vi "Variables Data IO.vi"(6 "Write blank data ?(F)":bool, 7 "Select":T1, 8 "error in":errorcluster caption="에러 입력(에러 없음)", 9 "Data In":string[][](array[string]), 11 "Func_ext":string) -> (0 "error out":errorcluster caption="에러 출력", 1 "Data Out":string[][](array[string]), 3 "Func_ext Out":string)   [LabVIEW 2020]
uses:
  Controls/Cmd_Var Data IO.ctl
  Variables/Global_Condition.vi
  Variables/Global_Resolution.vi
  Variables/Global_Spec.vi
  Variables/Global_Result.vi
  Variables/Global_STD.vi
  Variables/Global_CMC.vi
  Variables/Global_Cal Info.vi
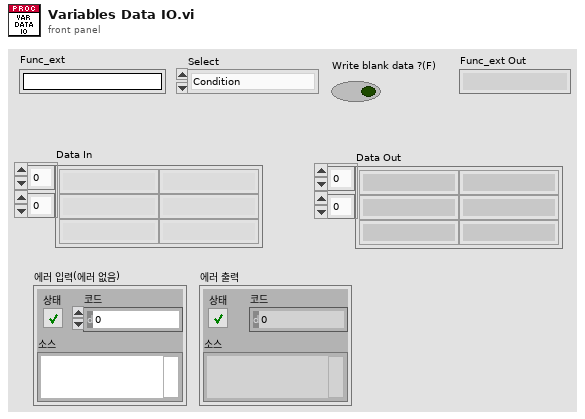
[diagram p1: front panel]
types:
  T1 = typedef "Cmd_Var Data IO.ctl" = enum16{"Condition", "Condition Default", "Condition_Temp", "Resolution", "Resolution Default", "Resolution Old", "Spec", "Spec Default", "Spec Old", "Spec Temp", "Result", "Result2", "Result3", "Result_Temp", "Result_ADJ", "Result_ADJ2", "STD1", "STD2", "STD3", "STD4", "STD5", "STD Temp", "CMC", "CMC Default"}
  T2 = cluster{"Func 0":string[][], "Func 1":string[][], "Func 2":string[][], "Func 3":string[][], "Func 4":string[][], "Func 5":string[][], "Func 6":string[][], "Func 7":string[][], "Func 8":string[][], "Func 9":string[][], "Func 10":string[][], "Func 11":string[][], "Func 12":string[][], "Func 13":string[][], "Func 14":string[][], "Func 15":string[][], "Func 16":string[][], "Func 17":string[][], "Func 18":string[][], "Func 19":string[][]}
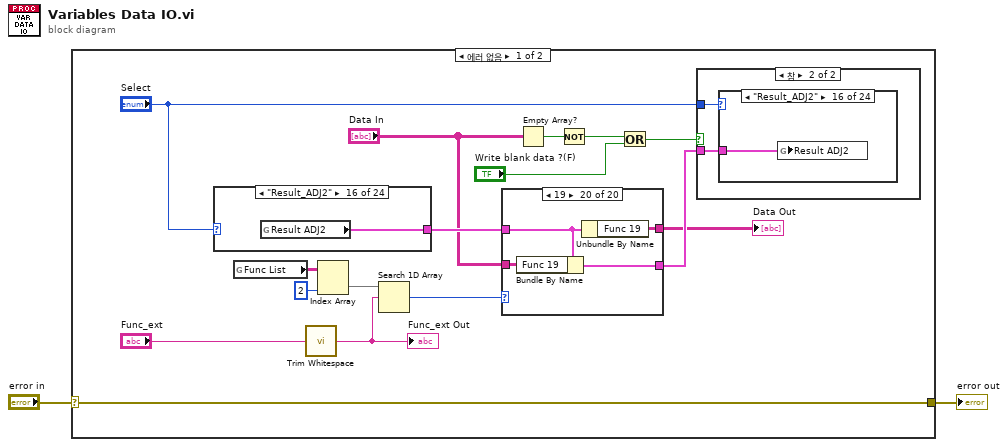
[diagram p0: block diagram]
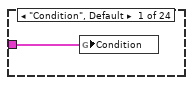
[diagram p3: hidden frame]
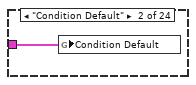
[diagram p4: hidden frame]
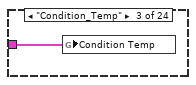
[diagram p5: hidden frame]
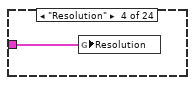
[diagram p6: hidden frame]
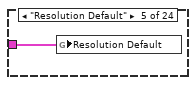
[diagram p7: hidden frame]
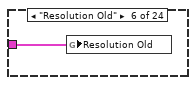
[diagram p8: hidden frame]
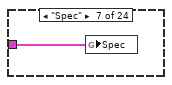
[diagram p9: hidden frame]
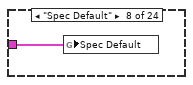
[diagram p10: hidden frame]
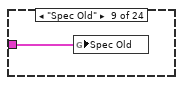
[diagram p11: hidden frame]
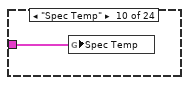
[diagram p12: hidden frame]
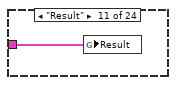
[diagram p13: hidden frame]
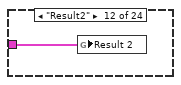
[diagram p14: hidden frame]
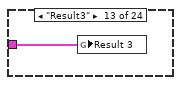
[diagram p15: hidden frame]
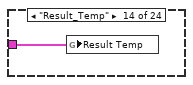
[diagram p16: hidden frame]
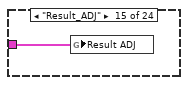
[diagram p17: hidden frame]
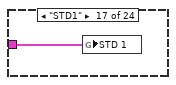
[diagram p18: hidden frame]
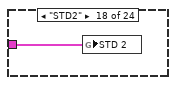
[diagram p19: hidden frame]
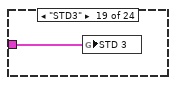
[diagram p20: hidden frame]
diagram:
  n1 = case shown="에러 없음" "error in" {
    selector: "error in" -> [w12 w149]
    tunnel: [w12 w149] -> w1
    frame No Error {
      n2 = case shown="\"Result_ADJ2\"" "Select" {
        tunnel: [w125 w126 w127 w128 w129 w130 w131 w132 w133 w134 w135 w136 w137 w138 w139 w140 w141 w142 w143 w144 w145 w146 w147 w148] -> w18
        frame "Condition", Default {
          n3 = global read "Global_Condition.vi" "Condition"() -> (w125:T2)
        }
        frame "Condition Default" {
          n4 = global read "Global_Condition.vi" "Condition Default"() -> (w126:T2)
        }
        frame "Condition_Temp" {
          n5 = global read "Global_Condition.vi" "Condition Temp"() -> (w127:T2)
        }
        frame "Resolution" {
          n6 = global read "Global_Resolution.vi" "Resolution"() -> (w128:T2)
        }
        frame "Resolution Default" {
          n7 = global read "Global_Resolution.vi" "Resolution Default"() -> (w129:T2)
        }
        frame "Resolution Old" {
          n8 = global read "Global_Resolution.vi" "Resolution Old"() -> (w130:T2)
        }
        frame "Spec" {
          n9 = global read "Global_Spec.vi" "Spec"() -> (w131:T2)
        }
        frame "Spec Default" {
          n10 = global read "Global_Spec.vi" "Spec Default"() -> (w132:T2)
        }
        frame "Spec Old" {
          n11 = global read "Global_Spec.vi" "Spec Old"() -> (w133:T2)
        }
        frame "Spec Temp" {
          n12 = global read "Global_Spec.vi" "Spec Temp"() -> (w134:T2)
        }
        frame "Result" {
          n13 = global read "Global_Result.vi" "Result"() -> (w135:T2)
        }
        frame "Result2" {
          n14 = global read "Global_Result.vi" "Result 2"() -> (w136:T2)
        }
        frame "Result3" {
          n15 = global read "Global_Result.vi" "Result 3"() -> (w137:T2)
        }
        frame "Result_Temp" {
          n16 = global read "Global_Result.vi" "Result Temp"() -> (w138:T2)
        }
        frame "Result_ADJ" {
          n17 = global read "Global_Result.vi" "Result ADJ"() -> (w139:T2)
        }
        frame "Result_ADJ2" {
          n18 = global read "Global_Result.vi" "Result ADJ2"() -> (w140:T2)
        }
        frame "STD1" {
          n19 = global read "Global_STD.vi" "STD 1"() -> (w141:T2)
        }
        frame "STD2" {
          n20 = global read "Global_STD.vi" "STD 2"() -> (w142:T2)
        }
        frame "STD3" {
          n21 = global read "Global_STD.vi" "STD 3"() -> (w143:T2)
        }
        frame "STD4" {
          n22 = global read "Global_STD.vi" "STD 4"() -> (w144:T2)
        }
        frame "STD5" {
          n23 = global read "Global_STD.vi" "STD 5"() -> (w145:T2)
        }
        frame "STD Temp" {
          n24 = global read "Global_STD.vi" "STD Temp"() -> (w146:T2)
        }
        frame "CMC" {
          n25 = global read "Global_CMC.vi" "CMC"() -> (w147:T2)
        }
        frame "CMC Default" {
          n26 = global read "Global_CMC.vi" "CMC Default"() -> (w148:T2)
        }
      }
      n27 = global read "Global_Cal Info.vi" "Func List"() -> (w6:string[][])
      n28 = call <vilib>:"Trim Whitespace.vi"("string"="Func_ext") -> ("trimmed string"=w3:string)  [unwired: 1 in]
      "Func_ext Out" <- w3
      n29 = Index Array(array=w6, index (col)=2 ("비활성화된 인덱스 (열)")) -> (element=w5:string[])  [unwired: 1 in]
      n30 = Search 1D Array(1D array=w5, element=w3) -> (index of element=w17:i32)  [unwired: 1 in]
      n31 = case shown="19" w17 {
        tunnel: w18 -> [w47 w51 w55 w59 w63 w67 w71 w75 w79 w83 w87 w91 w95 w99 w103 w107 w111 w115 w119 w123]
        tunnel: [w48 w52 w56 w60 w64 w68 w72 w76 w80 w84 w88 w92 w96 w100 w104 w108 w112 w116 w120 w124] -> w15
        tunnel: [w46 w50 w54 w58 w62 w66 w70 w74 w78 w82 w86 w90 w94 w98 w102 w106 w110 w114 w118 w122] -> w14
        tunnel: "Data In" -> [w45 w49 w53 w57 w61 w65 w69 w73 w77 w81 w85 w89 w93 w97 w101 w105 w109 w113 w117 w121]
        frame 0, Default {
          n32 = Bundle By Name(cluster=w47, "Func 0"=w45) -> (w48:T2)
          n33 = Unbundle By Name(w47) -> ("Func 0"=w46:string[][])
        }
        frame 1 {
          n34 = Bundle By Name(cluster=w51, "Func 1"=w49) -> (w52:T2)
          n35 = Unbundle By Name(w51) -> ("Func 1"=w50:string[][])
        }
        frame 2 {
          n36 = Bundle By Name(cluster=w55, "Func 2"=w53) -> (w56:T2)
          n37 = Unbundle By Name(w55) -> ("Func 2"=w54:string[][])
        }
        frame 3 {
          n38 = Bundle By Name(cluster=w59, "Func 3"=w57) -> (w60:T2)
          n39 = Unbundle By Name(w59) -> ("Func 3"=w58:string[][])
        }
        frame 4 {
          n40 = Bundle By Name(cluster=w63, "Func 4"=w61) -> (w64:T2)
          n41 = Unbundle By Name(w63) -> ("Func 4"=w62:string[][])
        }
        frame 5 {
          n42 = Bundle By Name(cluster=w67, "Func 5"=w65) -> (w68:T2)
          n43 = Unbundle By Name(w67) -> ("Func 5"=w66:string[][])
        }
        frame 6 {
          n44 = Bundle By Name(cluster=w71, "Func 6"=w69) -> (w72:T2)
          n45 = Unbundle By Name(w71) -> ("Func 6"=w70:string[][])
        }
        frame 7 {
          n46 = Bundle By Name(cluster=w75, "Func 7"=w73) -> (w76:T2)
          n47 = Unbundle By Name(w75) -> ("Func 7"=w74:string[][])
        }
        frame 8 {
          n48 = Bundle By Name(cluster=w79, "Func 8"=w77) -> (w80:T2)
          n49 = Unbundle By Name(w79) -> ("Func 8"=w78:string[][])
        }
        frame 9 {
          n50 = Bundle By Name(cluster=w83, "Func 9"=w81) -> (w84:T2)
          n51 = Unbundle By Name(w83) -> ("Func 9"=w82:string[][])
        }
        frame 10 {
          n52 = Bundle By Name(cluster=w87, "Func 10"=w85) -> (w88:T2)
          n53 = Unbundle By Name(w87) -> ("Func 10"=w86:string[][])
        }
        frame 11 {
          n54 = Bundle By Name(cluster=w91, "Func 11"=w89) -> (w92:T2)
          n55 = Unbundle By Name(w91) -> ("Func 11"=w90:string[][])
        }
        frame 12 {
          n56 = Bundle By Name(cluster=w95, "Func 12"=w93) -> (w96:T2)
          n57 = Unbundle By Name(w95) -> ("Func 12"=w94:string[][])
        }
        frame 13 {
          n58 = Bundle By Name(cluster=w99, "Func 13"=w97) -> (w100:T2)
          n59 = Unbundle By Name(w99) -> ("Func 13"=w98:string[][])
        }
        frame 14 {
          n60 = Bundle By Name(cluster=w103, "Func 14"=w101) -> (w104:T2)
          n61 = Unbundle By Name(w103) -> ("Func 14"=w102:string[][])
        }
        frame 15 {
          n62 = Bundle By Name(cluster=w107, "Func 15"=w105) -> (w108:T2)
          n63 = Unbundle By Name(w107) -> ("Func 15"=w106:string[][])
        }
        frame 16 {
          n64 = Bundle By Name(cluster=w111, "Func 16"=w109) -> (w112:T2)
          n65 = Unbundle By Name(w111) -> ("Func 16"=w110:string[][])
        }
        frame 17 {
          n66 = Bundle By Name(cluster=w115, "Func 17"=w113) -> (w116:T2)
          n67 = Unbundle By Name(w115) -> ("Func 17"=w114:string[][])
        }
        frame 18 {
          n68 = Bundle By Name(cluster=w119, "Func 18"=w117) -> (w120:T2)
          n69 = Unbundle By Name(w119) -> ("Func 18"=w118:string[][])
        }
        frame 19 {
          n70 = Bundle By Name(cluster=w123, "Func 19"=w121) -> (w124:T2)
          n71 = Unbundle By Name(w123) -> ("Func 19"=w122:string[][])
        }
      }
      "Data Out" <- w14
      n72 = Empty Array?(array="Data In") -> (empty?=w8:bool)
      n73 = Not(x=w8) -> (.not. x?=w7:bool)
      n74 = Or(x=w7, y="Write blank data ?(F)") -> (x .or. y?=w9:bool)
      n75 = case shown="참" w9 {
        tunnel: "Select" -> [_ w20]
        tunnel: w15 -> [_ w19]
        frame False {
        }
        frame True {
          n76 = case shown="\"Result_ADJ2\"" w20 {
            tunnel: w19 -> [w21 w22 w23 w24 w25 w26 w27 w28 w29 w30 w31 w32 w33 w34 w35 w36 w37 w38 w39 w40 w41 w42 w43 w44]
            frame "Condition", Default {
              n77 = global write "Global_Condition.vi" "Condition"(w21) -> ()
            }
            frame "Condition Default" {
              n78 = global write "Global_Condition.vi" "Condition Default"(w22) -> ()
            }
            frame "Condition_Temp" {
              n79 = global write "Global_Condition.vi" "Condition Temp"(w23) -> ()
            }
            frame "Resolution" {
              n80 = global write "Global_Resolution.vi" "Resolution"(w24) -> ()
            }
            frame "Resolution Default" {
              n81 = global write "Global_Resolution.vi" "Resolution Default"(w25) -> ()
            }
            frame "Resolution Old" {
              n82 = global write "Global_Resolution.vi" "Resolution Old"(w26) -> ()
            }
            frame "Spec" {
              n83 = global write "Global_Spec.vi" "Spec"(w27) -> ()
            }
            frame "Spec Default" {
              n84 = global write "Global_Spec.vi" "Spec Default"(w28) -> ()
            }
            frame "Spec Old" {
              n85 = global write "Global_Spec.vi" "Spec Old"(w29) -> ()
            }
            frame "Spec Temp" {
              n86 = global write "Global_Spec.vi" "Spec Temp"(w30) -> ()
            }
            frame "Result" {
              n87 = global write "Global_Result.vi" "Result"(w31) -> ()
            }
            frame "Result2" {
              n88 = global write "Global_Result.vi" "Result 2"(w32) -> ()
            }
            frame "Result3" {
              n89 = global write "Global_Result.vi" "Result 3"(w33) -> ()
            }
            frame "Result_Temp" {
              n90 = global write "Global_Result.vi" "Result Temp"(w34) -> ()
            }
            frame "Result_ADJ" {
              n91 = global write "Global_Result.vi" "Result ADJ"(w35) -> ()
            }
            frame "Result_ADJ2" {
              n92 = global write "Global_Result.vi" "Result ADJ2"(w36) -> ()
            }
            frame "STD1" {
              n93 = global write "Global_STD.vi" "STD 1"(w37) -> ()
            }
            frame "STD2" {
              n94 = global write "Global_STD.vi" "STD 2"(w38) -> ()
            }
            frame "STD3" {
              n95 = global write "Global_STD.vi" "STD 3"(w39) -> ()
            }
            frame "STD4" {
              n96 = global write "Global_STD.vi" "STD 4"(w40) -> ()
            }
            frame "STD5" {
              n97 = global write "Global_STD.vi" "STD 5"(w41) -> ()
            }
            frame "STD Temp" {
              n98 = global write "Global_STD.vi" "STD Temp"(w42) -> ()
            }
            frame "CMC" {
              n99 = global write "Global_CMC.vi" "CMC"(w43) -> ()
            }
            frame "CMC Default" {
              n100 = global write "Global_CMC.vi" "CMC Default"(w44) -> ()
            }
          }
        }
      }
    }
    frame Error {
    }
  }
  "error out" <- w1
